vi "OOB to Logic FGV.vi"(7 "Op (Get)":enum16{"Get", "Set"}(ring), 8 "error in (no error)":errorcluster, 11 "OOB to Logic Data in":T1) -> (0 "error out":errorcluster, 3 "OOB to Logic Data out":T1)   [LabVIEW 2025, in "OOB Data Transfer.lvlib"]
uses:
  OOB Data Transfer.lvlib
  Typdefs/OOB to Logic Data.ctl
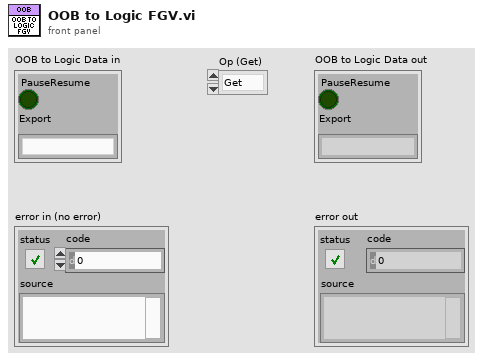
[diagram p1: front panel]
types:
  T1 = typedef "OOB Data Transfer.lvlib/OOB to Logic Data.ctl" = cluster{"PauseResume":bool, "Export":string}
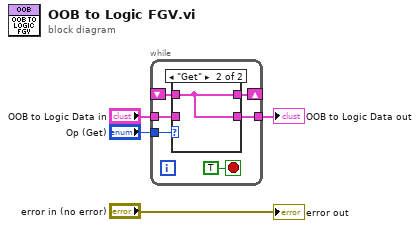
[diagram p0: block diagram]
diagram:
  n1 = while {
    tunnel: "Op (Get)" -> [w9]
    tunnel: "OOB to Logic Data in" -> [w8]
    shift-right: [w7] -> _
    shift-left: _ -> [w6]
    tunnel: [w5] -> w1
    stop <- TRUE stop-if-true
    n2 = case shown="\"Get\"" w9 {
      tunnel: w8 -> [w11 _]
      tunnel: [w11 w12] -> w7
      tunnel: [w11 w12] -> w5
      tunnel: w6 -> [_ w12]
      frame "Set" {
      }
      frame "Get" {
      }
    }
  }
  "OOB to Logic Data out" <- w1
  "error out" <- "error in (no error)"
